vi "Channel GUID.vi"() -> (3 "GUID":string="88fcfa75-3196-4ae9-a459-f2e46a72afc7")   [LabVIEW 2017, in "Data Sharing Framework System Explorer.lvlib"]
uses:
  Data Sharing Framework System Explorer.lvlib
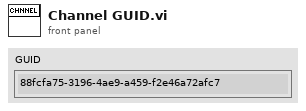
[diagram p1: front panel]
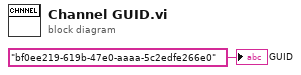
[diagram p0: block diagram]
diagram:
  "GUID" <- "bf0ee219-619b-47e0-aaaa-5c2edfe266e0" ("Data Sharing Framework")
